vi "Insight_RW_Number_of_Pts.vi"(7 "Parameter Type":enum16{"Value", "MAXimum", "MINimum", "DEFault"}(ring), 8 "error in (no error)":errorcluster, 9 "Mode (Read / Write)":enum8{"Write", "Read"}(ring), 10 "Number of Points":u32=2800, 11 "telnet connection":T1) -> (0 "error out":errorcluster, 1 "response data":string, 2 "Number of Points":u32, 3 "telnet  connection out":T1)   [LabVIEW 2014]
doc: "Insight Photonic Solutions\n\nThis VI reads or writes the Number of Points in the sweep of the laser.\n\nINPUTS\n\nMode - Tells the VI whether the command is a Read or a Write. (Default = Read).\nParameter Type - Tells the VI whether the command should use a Value or a keyword MAXimum, MINimum or DEFault to set the parameter value. (Default = Value).\nNumber of Points - The numeric value to set the number of points during a sweep. (Default = 2800).\nerror in - The standard LabView Error cluster. Use this to enforce sequentiality and error tracking.\n\nOUTPUTS\n\nresponse data - the complete response string from the laser\nNumber of Points - the number of points written to or read from the laser\nerror out - the standard error cluster. Reports errors in reading or writing to the laser, or passes through errors from before this VI.\n\nver 1.0 - original release\nver 1.1 - return full response string and capture errors if command or parameters not recognized.\nver 3.2 - parser handles responses from Atlas version 3.1 and earlier or version 3.2 and later.\nver 3.4 - allows writing and reading key values Max, Min or Default for the parameter"
uses:
  Telnet Session.ctl
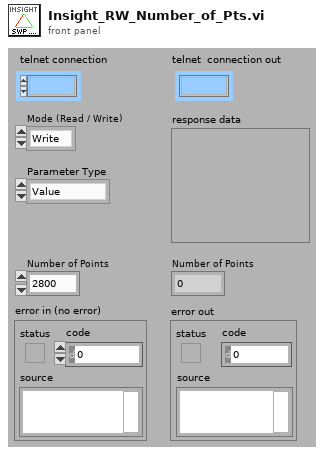
[diagram p1: front panel]
types:
  T1 = typedef "Telnet Session.ctl" = refnum<k1>
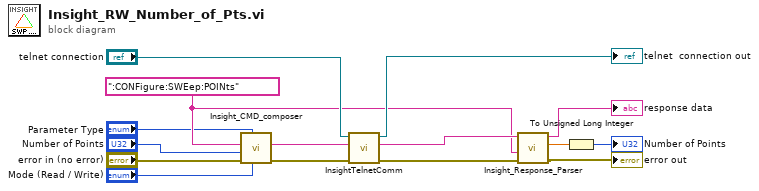
[diagram p0: block diagram]
diagram:
  w5 = ":CONFigure:SWEep:POINts" ("String")
  n1 = call "Insight_CMD_composer.vi"("Mode (Read / Write)"="Mode (Read / Write)", "Parameter Type"="Parameter Type", "error in (no error)"="error in (no error)", "Value"="Number of Points", "CMD"=w5) -> ("error out"=w7:errorcluster, "Command String"=w6:string)  [unwired: 5 in]
  n2 = call "InsightTelnetComm.vi"("error in"=w7, "write buffer (\"\")"=w6, "telnet connection"="telnet connection") -> ("error out"=w13:errorcluster, "response data"=w12:string, "telnet  connection out"=→"telnet  connection out":T1)  [unwired: 4 in]
  n3 = call "Insight_Response_Parser.vi"("error in (no error)"=w13, "Command String"=w5, "Laser Response In"=w12) -> ("error out"=→"error out":errorcluster, "Value"=w9:dbl, "Laser Response Out"=→"response data":string)  [unwired: 6 in]
  n4 = To Unsigned Long Integer(number=w9) -> (unsigned 32bit integer=→"Number of Points":u32)
